vi "初级扫雷.vi"() -> ()   [LabVIEW 2014]
panel:
  in  "列":i32
  in  "雷":i32
  in  "行":i32
  out "提示":i16[][](array[numeric])
  out "数组 3":i32[][](array[ring])
  # "：）"
  # "扫雷\n注：\n1、完全自定义，请在开始前设置参数，请合理设置参数。\n2、右键插小旗。\n3、单次执行时，游戏成功或是失败都会结束程序。\n4、点击是依靠坐标，请千万不要移动显示数组的位置，\n   保持左上角与O点重合。\n\n向右看，有答案————————>>>>"
  # "O"
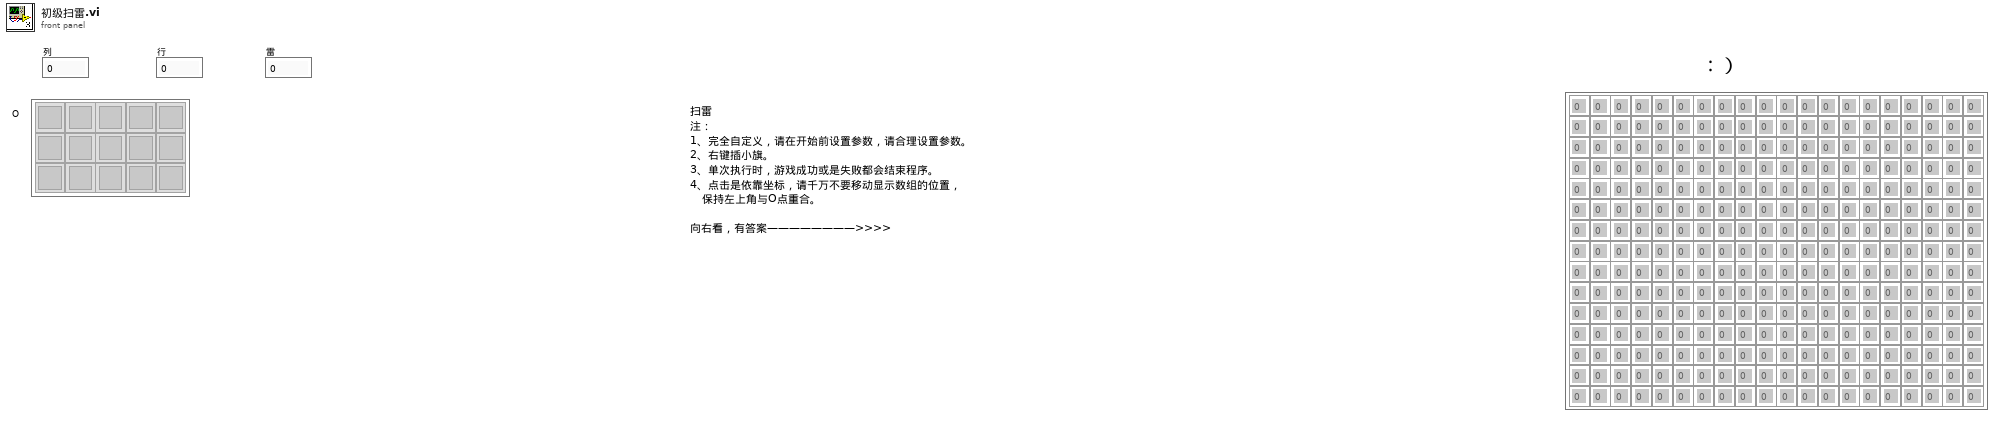
[diagram p1: front panel]
types:
  T1 = typedef "LVPoint32TypeDef.ctl" = cluster{"Horizontal":i32, "Vertical":i32}
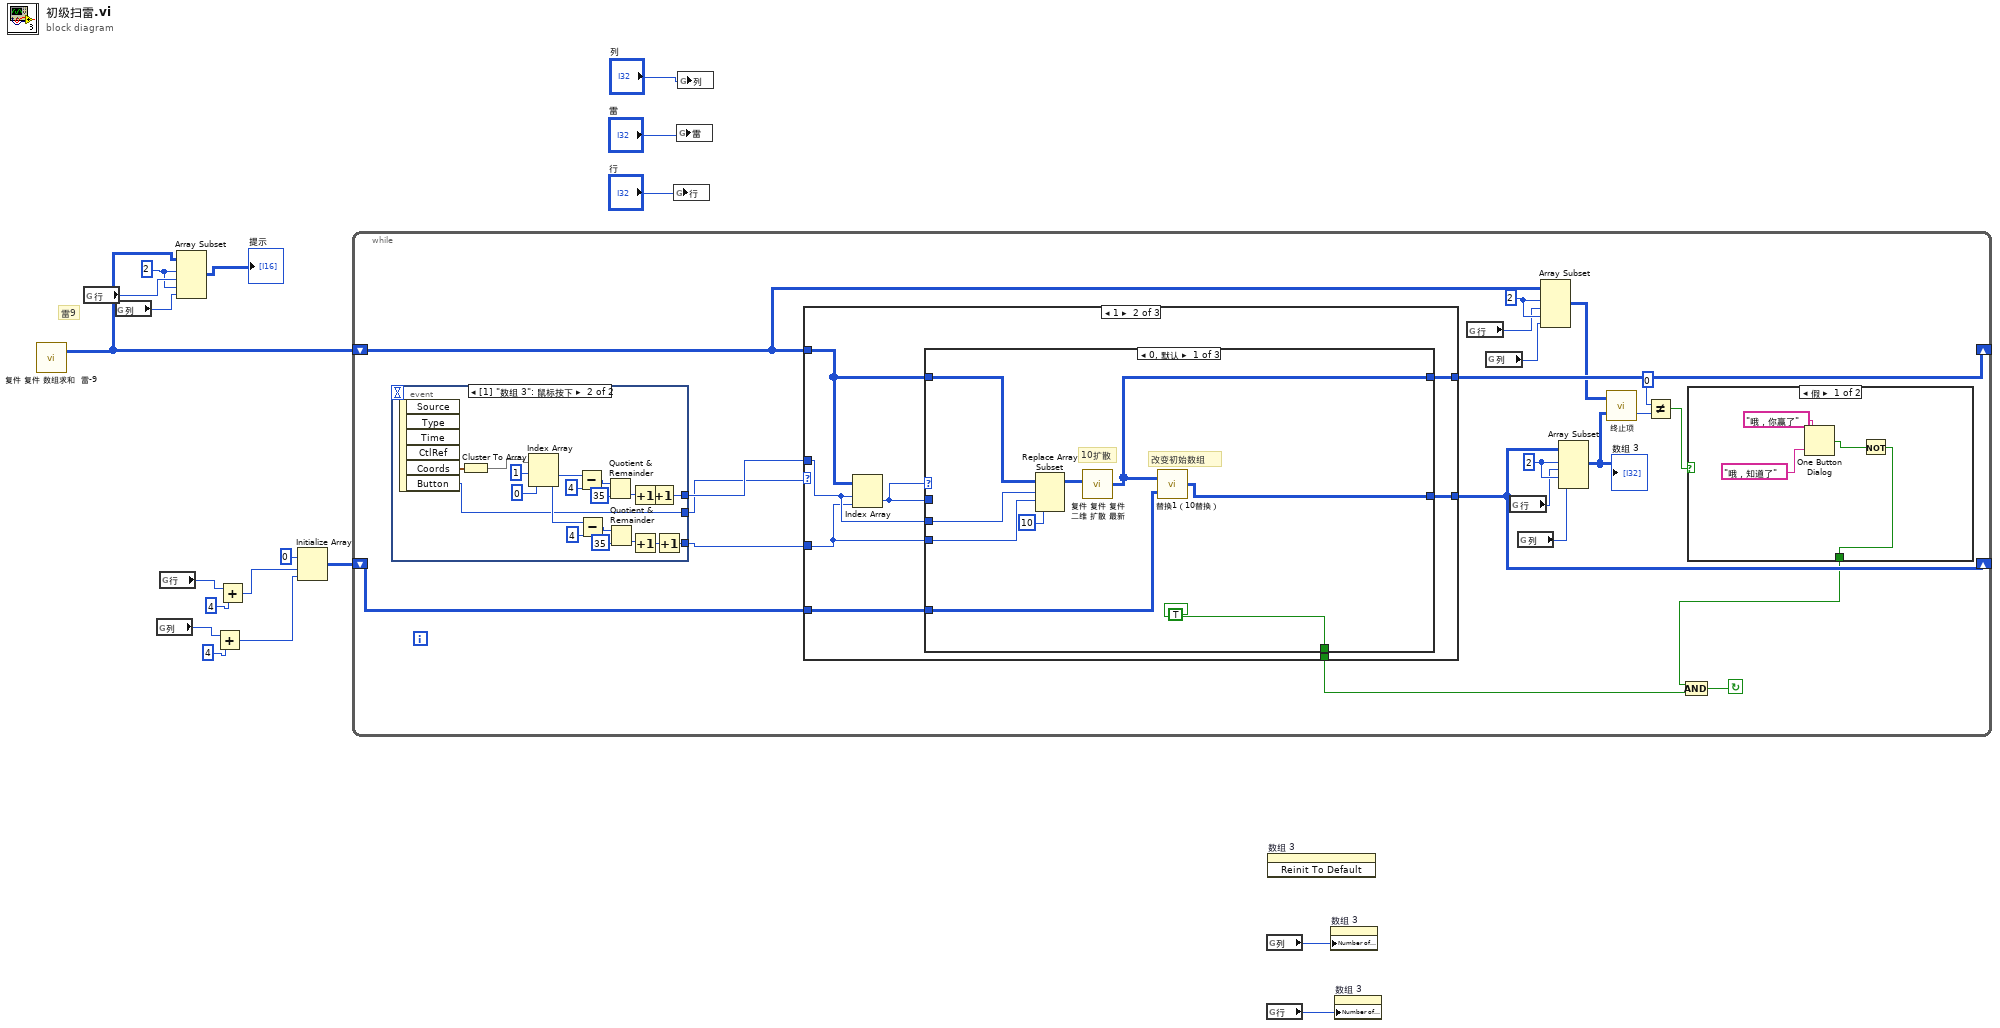
[diagram p0: block diagram]
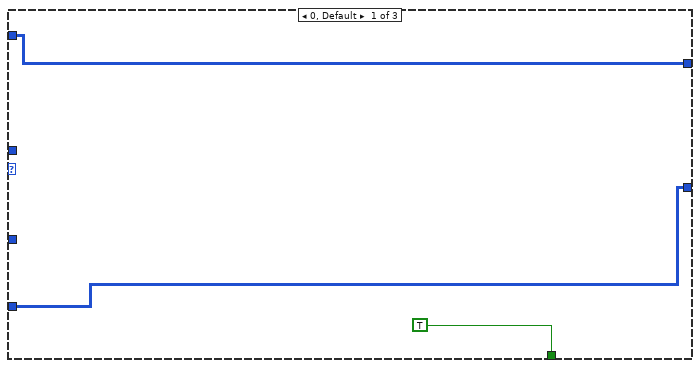
[diagram p3: hidden frame]
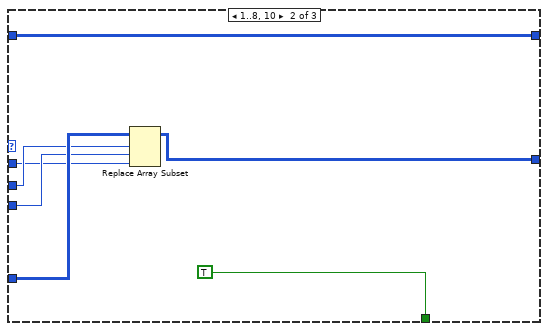
[diagram p4: hidden frame]
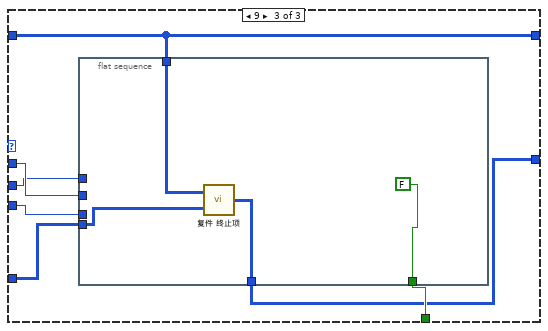
[diagram p5: hidden frame]
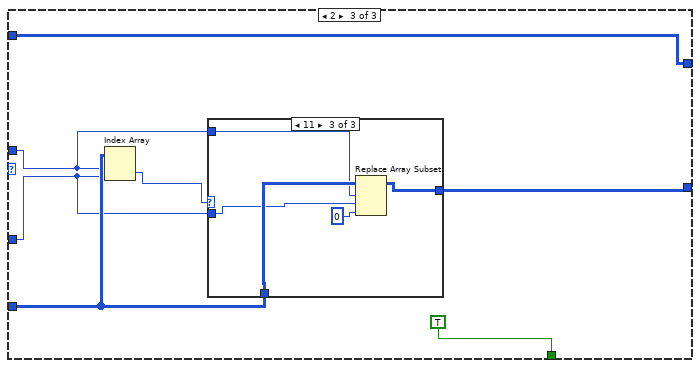
[diagram p6: hidden frame]
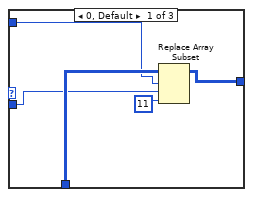
[diagram p7: hidden frame]
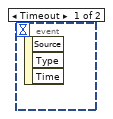
[diagram p9: hidden frame]
diagram:
  w5 = 2
  # "雷9"
  n1 = call "复件 复件 数组求和  雷-9.vi"() -> ("数组 2"=w11:i16[][])
  n2 = global read "全局 1.vi" "行"() -> (w6:i32)
  n3 = global read "全局 1.vi" "列"() -> (w4:i32)
  n4 = global read "全局 1.vi" "列"() -> (w2:i32)
  n5 = global read "全局 1.vi" "行"() -> (w8:i32)
  n6 = Array Subset(array=w11, index (row)=w5, length (row)=w6, index (col)=w5, length (col)=w4) -> (→"提示":i16[][])
  n7 = Add(x=w2, y=4) -> (x+y=w1:i32)
  n8 = Add(x=w8, y=4) -> (x+y=w7:i32)
  n9 = Initialize Array(0, w7, w1) -> (w12:i32[][])
  n10 = while {
    shift-right: [w37] -> _
    shift-left: w12 -> [w39]
    shift-right: [w38] -> _
    shift-left: w11 -> [w36]
    stop <- w21 continue-if-true
    w29 = 2
    w32 = 2
    n11 = event shown="[1] \"数组 3\": 鼠标按下" {
      selector: _ -> [_ _]
      dyn-events: _ -> [_ _]
      timeout: _ -> [_ _]
      tunnel: [_ w102] -> w35
      tunnel: [_ w101] -> w34
      tunnel: [_ w105] -> w24
      event Timeout {
        n12 = event-data() -> ()  [unwired: 1 in, 3 out]
      }
      event "数组 3": Mouse Down {
        n13 = event-data() -> ("Coords"=w103:T1, "Button"=w105:u16)  [unwired: 1 in, 4 out]
        n14 = Cluster To Array(cluster=w103) -> (array=w104:i32[])
        n15 = Index Array(array=w104, index #1=1, index #2=0) -> (element #1=w115:i32, element #2=w110:i32)
        n16 = Subtract(x=w115, y=4) -> (x-y=w117:i32)
        n17 = Subtract(x=w110, y=4) -> (x-y=w113:i32)
        n18 = Quotient & Remainder(x=w117, y=35) -> (floor(x/y)=w109:i32)  [unwired: 1 out]
        n19 = Quotient & Remainder(x=w113, y=35) -> (floor(x/y)=w108:i32)  [unwired: 1 out]
        n20 = Increment(x=w109) -> (x+1=w107:i32)
        n21 = Increment(x=w108) -> (x+1=w106:i32)
        n22 = Increment(x=w107) -> (x+1=w102:i32)
        n23 = Increment(x=w106) -> (x+1=w101:i32)
      }
    }
    n24 = case shown="1" w24 {
      tunnel: w39 -> [w46 w55 w86]
      tunnel: [w47 w54 w89] -> w38
      tunnel: [w46 w53 w87] -> w37
      tunnel: w36 -> [w47 w52 w89]
      tunnel: w35 -> [_ w51 w85]
      tunnel: w34 -> [_ w50 w84]
      tunnel: [TRUE w48 TRUE] -> w30
      frame 0, Default {
      }
      frame 1 {
        n25 = Index Array(array=w52, index (row)=w51, index (col)=w50) -> (element=w49:i32)
        n26 = case shown="0, 默认" w49 {
          tunnel: w52 -> [w64 w66 w73]
          tunnel: w51 -> [w62 w70 w76]
          tunnel: w50 -> [w61 w69 w75]
          tunnel: [w58 w67 w72] -> w53
          tunnel: w55 -> [w59 w71 w78]
          tunnel: w49 -> [_ w68 w77]
          tunnel: [w57 w66 w73] -> w54
          tunnel: [TRUE TRUE w74] -> w48
          frame 0, Default {
            # "改变初始数组"
            # "10扩散"
            n27 = Replace Array Subset(array=w64, new element=10, index (row)=w62, index (col)=w61) -> (w63:i32[][])
            n28 = call "复件 复件 复件 二维 扩散 最新.vi"("数组 2"=w63) -> ("数组"=w57:i32[][])
            n29 = call "替换1（10替换）.vi"("改变的数组"=w59, "检索的数组"=w57) -> ("显示 2"=w58:i32[][])
          }
          frame 1..8, 10 {
            n30 = Replace Array Subset(array=w71, new element=w68, index (row)=w70, index (col)=w69) -> (w67:i32[][])
          }
          frame 9 {
            n31 = flat-sequence {
              tunnel: [FALSE] -> w74
              tunnel: [w80] -> w72
              tunnel: w73 -> [w81]
              tunnel: w75 -> [_]
              tunnel: w76 -> [_]
              tunnel: w77 -> [_]
              tunnel: w78 -> [w82]
              frame #0 {
                n32 = call "复件 终止项.vi"("结果"=w82, "检索"=w81) -> ("结果 2"=w80:i32[][])
              }
            }
          }
        }
      }
      frame 2 {
        n33 = Index Array(array=w86, index (row)=w85, index (col)=w84) -> (element=w83:i32)
        n34 = case shown="11" w83 {
          tunnel: [w93 w95 w96] -> w87
          tunnel: w86 -> [w92 w95 w99]
          tunnel: w85 -> [w91 _ w97]
          tunnel: w84 -> [w90 _ w98]
          frame 0, Default {
            n35 = Replace Array Subset(array=w92, new element=11, index (row)=w91, index (col)=w90) -> (w93:i32[][])
          }
          frame 1..10 {
          }
          frame 11 {
            n36 = Replace Array Subset(array=w99, new element=0, index (row)=w97, index (col)=w98) -> (w96:i32[][])
          }
        }
      }
    }
    n37 = global read "全局 1.vi" "行"() -> (w26:i32)
    n38 = global read "全局 1.vi" "列"() -> (w23:i32)
    n39 = global read "全局 1.vi" "行"() -> (w25:i32)
    n40 = global read "全局 1.vi" "列"() -> (w22:i32)
    n41 = Array Subset(array=w36, index (row)=w29, length (row)=w26, index (col)=w29, length (col)=w23) -> (w28:i32[][])
    n42 = Array Subset(array=w37, index (row)=w32, length (row)=w25, index (col)=w32, length (col)=w22) -> (w33:i32[][])
    "数组 3" <- w33
    n43 = call "终止项.vi"("结果"=w33, "检索"=w28) -> ("数值"=w31:i32)
    n44 = Not Equal?(x=0, y=w31) -> (x != y?=w20:bool)
    n45 = case shown="假" w20 {
      selector: w20 -> [_ w44]
      tunnel: [w40 w44] -> w19
      frame False {
        n46 = One Button Dialog(message="哦，你赢了", button name ("OK")="哦，知道了") -> (true=w41:bool)
        n47 = Not(x=w41) -> (.not. x?=w40:bool)
      }
      frame True {
      }
    }
    n48 = And(x=w19, y=w30) -> (x .and. y?=w21:bool)
  }
  n49 = global write "全局 1.vi" "行"("行") -> ()
  n50 = global write "全局 1.vi" "雷"("雷") -> ()
  n51 = global write "全局 1.vi" "列"("列") -> ()
  n52 = global read "全局 1.vi" "列"() -> (w15:i32)
  n53 = global read "全局 1.vi" "行"() -> (w14:i32)
  n54 = invoke on="数组 3" class="Arr (严格)" method="Reinit To Default"() -> ()  [unwired: 3 in, 3 out]
  n55 = property on="数组 3" class="Arr (严格)"("Number of Columns"=w15) -> ()  [unwired: 2 in, 2 out]
  n56 = property on="数组 3" class="Arr (严格)"("Number of Rows"=w14) -> ()  [unwired: 2 in, 2 out]
